vi "Vision Research Phantom Series PhCon PhSetCineParams.vi"(0 "CN in":u32, 1 "Cine":T1=-2 items=["CINE_DEFAULT "=-2, "CINE_CURRENT "=-1, "CINE_PREVIEW  "=0, "CINE_FIRST    "=1, "FIRST_FLASH_CINE"=101], 3 "ACQUIPARAMS":T2 {"CFA"."CFA" items=["CFA_NONE", "CFA_VRI", "CFA_VRIV6", "CFA_BAYER", "CFA_BAYERFLIP"]; "TriggerTime"."fractions" format="%32.0f"}, 5 "Error In (no error)":errorcluster) -> (14 "CN out":u32=1, 15 "Cine out":T1=-2 items=["CINE_DEFAULT "=-2, "CINE_CURRENT "=-1, "CINE_PREVIEW  "=0, "CINE_FIRST    "=1, "FIRST_FLASH_CINE"=101], 17 "ACQUIPARAMS out":T2 {"CFA"."CFA" items=["CFA_NONE", "CFA_VRI", "CFA_VRIV6", "CFA_BAYER", "CFA_BAYERFLIP"]; "TriggerTime"."fractions" format="%32.0f"}, 19 "Error Out":errorcluster)   [LabVIEW 2013, in "VRI.lvlib"]
doc: "PhCon.dll\n\nPhSetCineParams\nHRESULT PhSetCineParams(UINT CN, INT Cine, PACQUIPARAMS pAcquiParams);\n\nParameters Description\nCN (in) Camera number.\nCine (in) Cine number.\npAcquiParams(in,out) The parameters to set. After the call you have in\n pAcquiParams the adjusted parameters; the out of \n range parameters will be changed to the nearest \n acceptable values.\nReturn HRESULT (0=Ok)\nComments Check and set the acquisition parameters. The order of\n checks is:\n 1. verify that the image dimensions are acceptable for \n this camera. If not, use the maximum dimensions.\n 2. Compute the maximum and the minimum frame rate \n for these dimensions and limit the FrameRate to \n this range.\n 3. Compute the maximum and the minimum exposure for\n this FrameRate and limit the Exposure to this range.\n 4. EDRExposure should be smaller than Exposure.\n 5. PTFrames and ImDelay should be non-zero.\n\nWritten by:\nBLOOMY CONTROLS, INC\nWINDSOR, CT 06095, USA\n860-298-9925\nwww.bloomy.com\nV1.0.0\nMay, 2004"
uses:
  VRI.lvlib
  _Type Defs/PhCon Predefined Cines.ctl
  _Type Defs/PHCon ACQUIPARAMS.ctl
  _Type Defs/PhCon SyncImaging.ctl
  _Type Defs/Rect.ctl
  _Type Defs/PHCon Time64.ctl
  _Type Defs/PhInt CFA.ctl
  Phantom DLLs/PhCon.dll
panel:
  # "For instructions on the use of this VI, press Ctrl+H to display the help window and move the mouse over the icon, controls, and indicators"
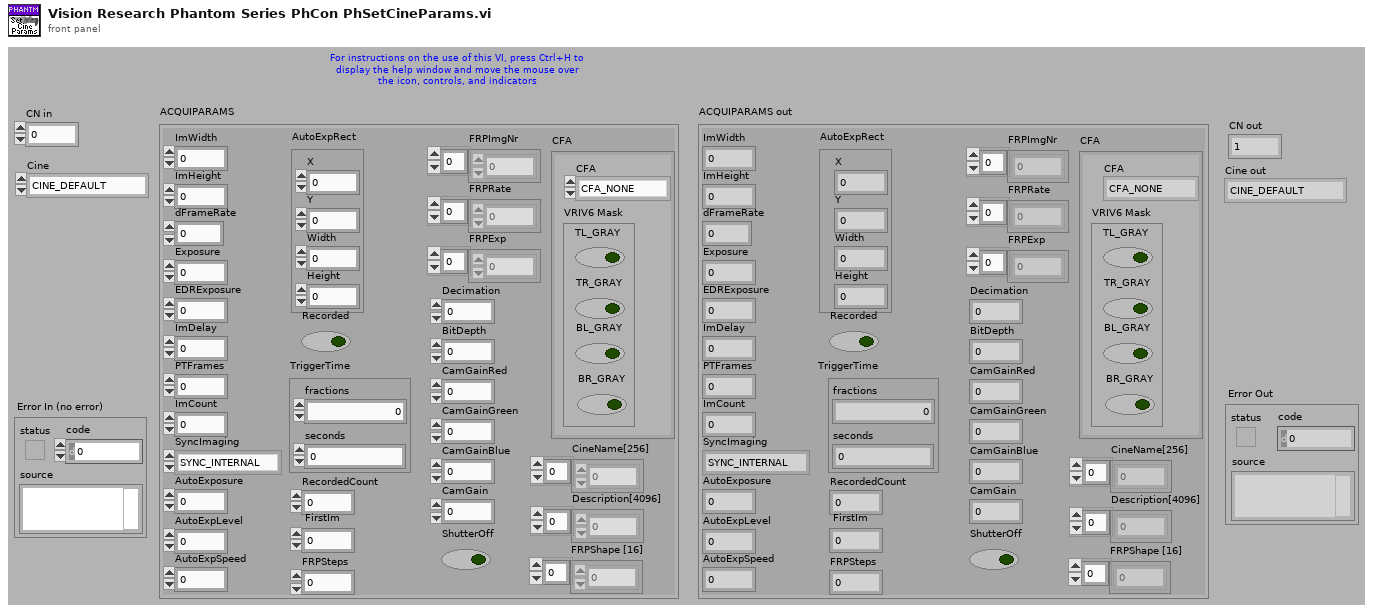
[diagram p1: front panel]
types:
  T1 = typedef "VRI.lvlib/PhCon Predefined Cines.ctl" = i32
  T2 = typedef "VRI.lvlib/PHCon ACQUIPARAMS.ctl" = cluster{"ImWidth":u32, "ImHeight":u32, "(deprecated)FrameRateInt":u32, "Exposure":u32, "EDRExposure":u32, "ImDelay":u32, "PTFrames":u32, "ImCount":u32, "SyncImaging":T3, "AutoExposure":u32, "AutoExpLevel":u32, "AutoExpSpeed":u32, "AutoExpRect":T4, "Recorded":bool, "TriggerTime":T5, "RecordedCount":u32, "FirstIm":i32, "FRPSteps":u32, "FRPImgNr":i32[], "FRPRate":u32[], "FRPExp":u32[], "Decimation":u32, "BitDepth":u32, "CamGainRed":u32, "CamGainGreen":u32, "CamGainBlue":u32, "CamGain":u32, "ShutterOff":bool, "CFA":T6, "CineName[256]":u8[], "Description[4096]":u8[], "FRPShape [16]":u32[], "dFrameRate":dbl}
  T3 = typedef "VRI.lvlib/PhCon SyncImaging.ctl" = enum32{"SYNC_INTERNAL", "SYNC_EXTERNAL", "SYNC_LOCKTOIRIG"}
  T4 = typedef "VRI.lvlib/Rect.ctl" = cluster{"X":i32, "Y":i32, "Width":i32, "Height":i32}
  T5 = typedef "VRI.lvlib/PHCon Time64.ctl" = cluster{"fractions":u32, "seconds":u32}
  T6 = typedef "VRI.lvlib/PhInt CFA.ctl" = cluster{"CFA":u32, "VRIV6 Mask":cluster{"TL_GRAY":bool, "TR_GRAY":bool, "BL_GRAY":bool, "BR_GRAY":bool}}
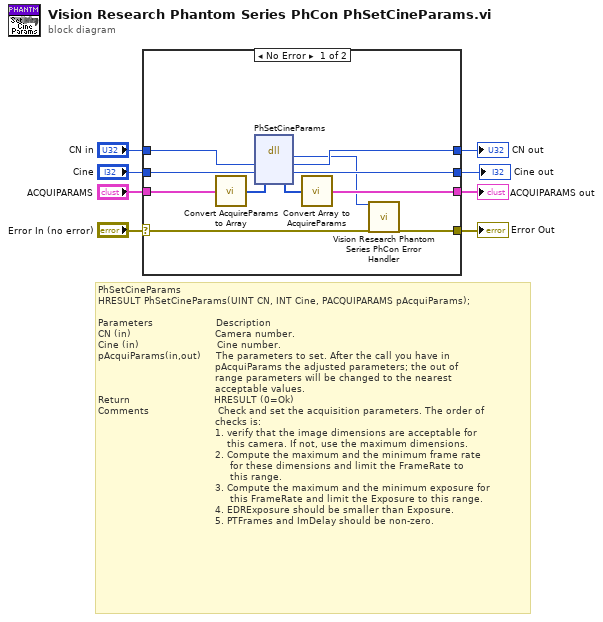
[diagram p0: block diagram]
diagram:
  # "PhSetCineParams\nHRESULT PhSetCineParams(UINT CN, INT Cine, PACQUIPARAMS pAcquiParams);\n\nParameters                     Description\nCN (in)                            Camera number.\nCine (in)                          Cine number.\npAcquiParams(in,out)     The parameters to set. After the call you have in\n                                       pAcquiParams the adjusted parameters; the out of \n                                       range parameters will be changed to the nearest \n                                       acceptable values.\nReturn                            HRESULT (0=Ok)\nComments                       Check and set the acquisition parameters. The order of\n                                       checks is:\n                                       1. verify that the image dimensions are acceptable for \n                                           this camera. If not, use the maximum dimensions.\n                                       2. Compute the maximum and the minimum frame rate \n                                            for these dimensions and limit the FrameRate to \n                                            this range.\n                                       3. Compute the maximum and the minimum exposure for\n                                            this FrameRate and limit the Exposure to this range.\n                                       4. EDRExposure should be smaller than Exposure.\n                                       5. PTFrames and ImDelay should be non-zero."
  n1 = case shown="No Error" "Error In (no error)" {
    selector: "Error In (no error)" -> [w19 w23]
    tunnel: [w18 w23] -> w7
    tunnel: "CN in" -> [w17 w22]
    tunnel: [w16 w22] -> w5
    tunnel: "Cine" -> [w15 w20]
    tunnel: "ACQUIPARAMS" -> [w14 w21]
    tunnel: [w13 w21] -> w2
    tunnel: [w12 w20] -> w1
    frame No Error {
      n2 = call "Convert AcquireParams to Array.vi"("ACQUIPARAMS"=w14) -> ("ACQUIPARAMS Data Array"=w10:u32[])
      n3 = dll-call lib="C:/Projects/SDK/32-bit/Vision Research Phantom Series Labview Driver/Phantom DLLs/PhCon.dll" fn="PhSetCineParams"("CN"=w17, "Cine"=w15, "pAcquiParams"=w10) -> ("HRESULT"=w11:i32, "CN"=w16:u32, "Cine"=w12:i32, "pAcquiParams"=w9:u32[])  [unwired: 3 in, 2 out]
      n4 = call "Convert Array to AcquireParams.vi"("ACQUIPARAMS BYTE ARRAY"=w9) -> ("ACQUIPARAMS"=w13:T2)
      n5 = call "Vision Research Phantom Series PhCon Error Handler.vi"("ErrNo"=w11, "Error In (no error)"=w19) -> ("Error Out"=w18:errorcluster)  [unwired: 17 out]
    }
    frame Error {
    }
  }
  "Error Out" <- w7
  "CN out" <- w5
  "ACQUIPARAMS out" <- w2
  "Cine out" <- w1
